vi "Generate header file text content.vi"(11 "header file template":T1) -> (3 "header file content":string)   [LabVIEW 2019, in "LabVIEW RGB565 Convertor.lvlib"]
uses:
  LabVIEW RGB565 Convertor.lvlib
  def-header file template.ctl
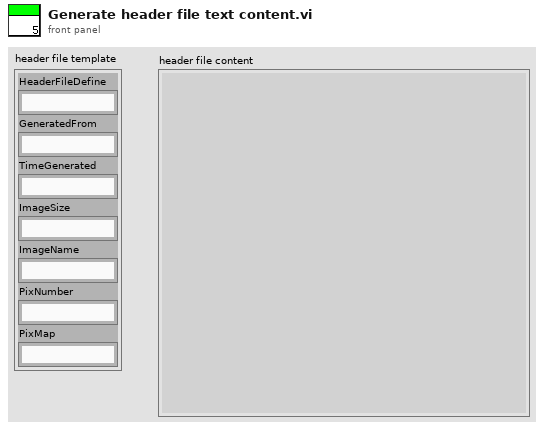
[diagram p1: front panel]
types:
  T1 = typedef "LabVIEW RGB565 Convertor.lvlib/def-header file template.ctl" = cluster{"HeaderFileDefine":string, "GeneratedFrom":string, "TimeGenerated":string, "ImageSize":string, "ImageName":string, "PixNumber":string, "PixMap":string}
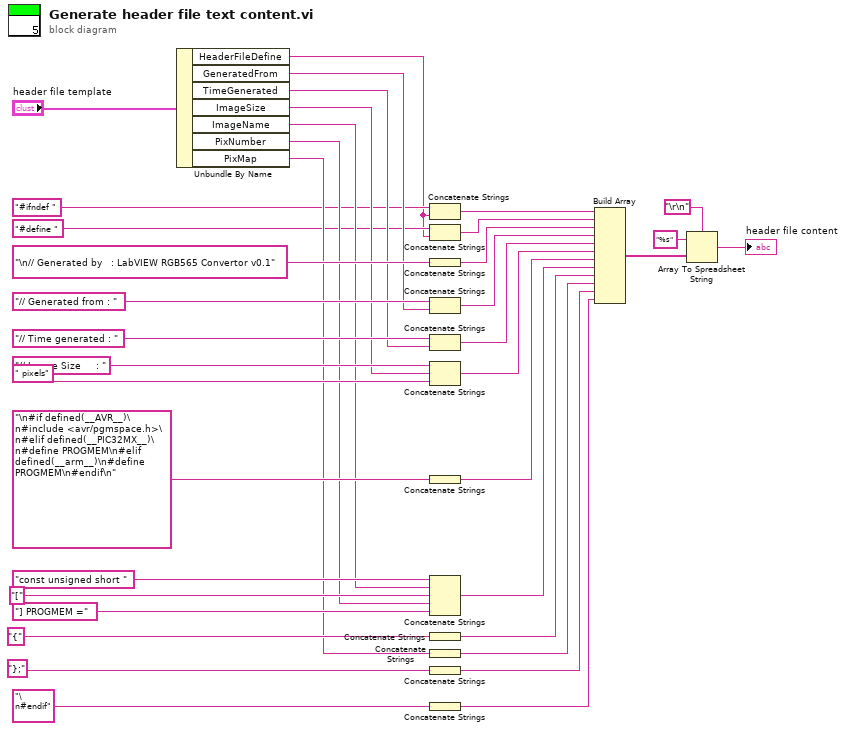
[diagram p0: block diagram]
diagram:
  n1 = Unbundle By Name("header file template") -> ("HeaderFileDefine"=w3:string, "GeneratedFrom"=w17:string, "TimeGenerated"=w16:string, "ImageSize"=w15:string, "ImageName"=w14:string, "PixNumber"=w13:string, "PixMap"=w12:string)
  n2 = Concatenate Strings("#ifndef " ("string"), w3) -> (w2:string)
  n3 = Concatenate Strings("#define " ("string"), w3) -> (w1:string)
  n4 = Concatenate Strings("\n// Generated by   : LabVIEW RGB565 Convertor v0.1" ("string")) -> (w30:string)
  n5 = Concatenate Strings("// Generated from : " ("string"), w17) -> (w31:string)
  n6 = Concatenate Strings("// Time generated : " ("string"), w16) -> (w32:string)
  n7 = Concatenate Strings("// Image Size     : " ("string"), w15, " pixels" ("string")) -> (w33:string)
  n8 = Concatenate Strings("\n#if defined(__AVR__)\n#include <avr/pgmspace.h>\n#elif defined(__PIC32MX__)\n#define PROGMEM\n#elif defined(__arm__)\n#define PROGMEM\n#endif\n" ("string")) -> (w34:string)
  n9 = Concatenate Strings("const unsigned short " ("string"), w14, "[" ("string"), w13, "] PROGMEM =" ("string")) -> (w35:string)
  n10 = Concatenate Strings("{" ("string")) -> (w36:string)
  n11 = Concatenate Strings(w12) -> (w37:string)
  n12 = Concatenate Strings("};" ("string")) -> (w38:string)
  n13 = Concatenate Strings("\n#endif" ("string")) -> (w6:string)
  n14 = Build Array(w2, w1, w30, w31, w32, w33, w34, w35, w36, w37, w38, w6) -> (w11:string[])
  n15 = Array To Spreadsheet String(delimiter (Tab)="\r\n", array=w11, 3:"%s" ("format string")) -> (spreadsheet string=→"header file content":string)
